vi "runtimeTest.vi"() -> ()   [LabVIEW 2017, in "JSON_RPC_Interface tests.lvlib"]
uses:
  JSON_RPC_Interface tests.lvlib
  module/execution/JSON_RPC_Interface runtime.lvclass
  <vilib>/NI/Tag Bus/dictionary/data dictionary.lvclass/data dictionary.ctl
  <vilib>/NI/Tag Bus/dictionary/lookup polymorphs/locate double.vi
  <vilib>/NI/Tag Bus/dictionary/lookup polymorphs/locate Array of String.vi
  <vilib>/NI/Tag Bus/table/data polymorphs/write one/write Double.vi
  <vilib>/NI/Tag Bus/table/data polymorphs/write one/write Array of String.vi
  <vilib>/NI/Tag Bus/table/data polymorphs/read one/read Double.vi
  <vilib>/NI/Tag Bus/table/data polymorphs/read one/read Array of String.vi
  <vilib>/NI/Tag Bus/dictionary/search/find data index.vi
  <vilib>/NI/Tag Bus/dictionary/search/search string list.vi
  module/configuration/JSON_RPC_Interface configuration.lvclass
  C:/Program Files (x86)/National Instruments/LabVIEW 2017/vi.lib/NI/Tag Bus Module Framework/module configuration/TBM module configuration.lvclass
  <vilib>/NI/Tag Bus/dictionary/tag not found.vi
  <vilib>/NI/Tag Bus/dictionary/data dictionary.lvclass
  <vilib>/NI/Tag Bus/table/data table.lvlib
panel:
  out "Input ArrayOfString":string[](array[string])
  in  "Output ArrayOfString":string[](array[string])
  in  "stop":bool
  in  "output value":dbl=42.0 format="%#_13g"
  out "Input value":dbl
  out "Names":string[](array[string])
  out "final error":errorcluster
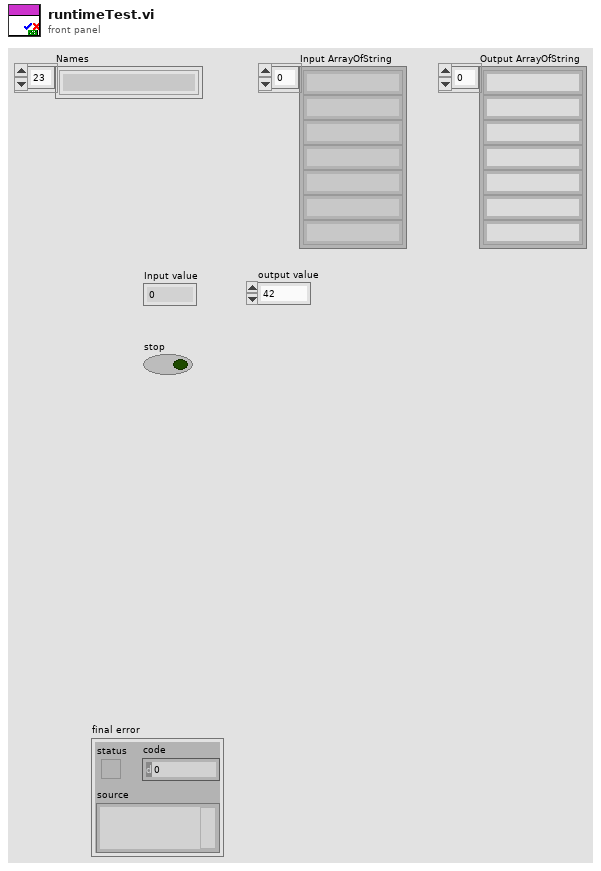
[diagram p1: front panel]
types:
  T1 = typedef "TBM channel.lvclass/data tables.ctl" = cluster{"input data":T2, "processing parameter":T2, "processing result":T2, "output data":T2}
  T2 = typedef "tag bus.lvlib/dictionary table pair.ctl" = cluster{"data dictionary":refnum<class "data dictionary.lvclass">, "data table":T3}
  T3 = typedef "tag bus.lvlib/data table.lvlib/data table.ctl" = cluster{"Double":dbl[], "Single":sgl[], "I64":i64[], "I32":i32[], "I16":i16[], "I8":i8[], "U64":u64[], "U32":u32[], "U16":u16[], "U8":u8[], "Boolean":bool[], "String":string[], "Array of Double":cluster{"DBL Array":dbl[]}[], "Array of Single":cluster{"SGL Array":sgl[]}[], "Array of I64":cluster{"I64 Array":i64[]}[], "Array of I32":cluster{"I32 Array":i32[]}[], "Array of I16":cluster{"I16 Array":i16[]}[], "Array of I8":cluster{"I8 Array":i8[]}[], "Array of U64":cluster{"U64 Array":u64[]}[], "Array of U32":cluster{"U32 Array":u32[]}[], "Array of U16":cluster{"U16 Array":u16[]}[], "Array of U8":cluster{"U8 Array":u8[]}[], "Array of Boolean":cluster{"Boolean Array":bool[]}[], "Array of String":cluster{"String Array":string[]}[]}
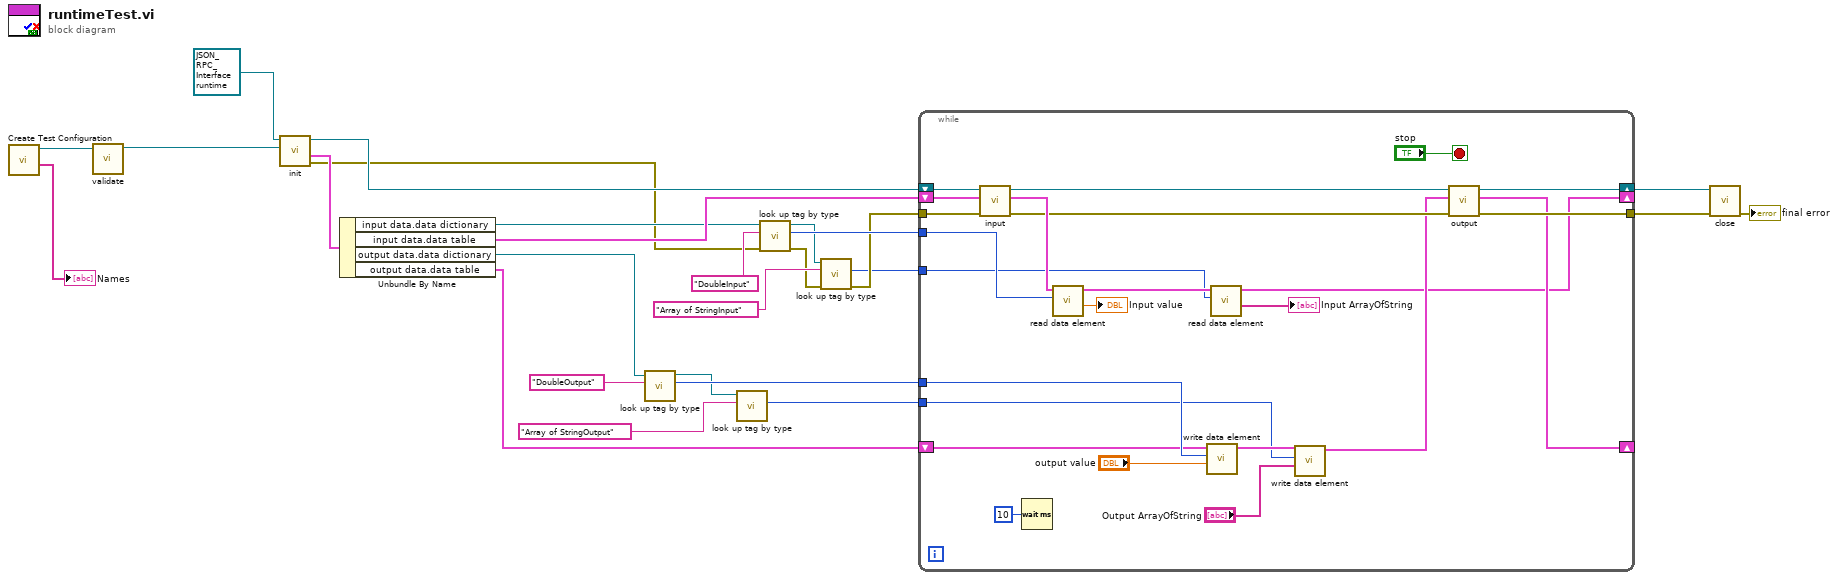
[diagram p0: block diagram]
diagram:
  n1 = call "Create Test Configuration.vi"() -> ("Names"=→"Names":string[], "Module Configuration"=w24:refnum<class "JSON_RPC_Interface configuration.lvclass">)  [unwired: 6 in, 4 out]
  n2 = call-dynamic "validate.vi"("JSON_RPC_Interface configuration in"=w24) -> ("JSON_RPC_Interface configuration out"=w25:refnum<class "JSON_RPC_Interface configuration.lvclass">)  [unwired: 9 in, 1 out]
  n3 = call-dynamic "init.vi"("TBM module configuration in"=w25, "JSON_RPC_Interface runtime in"=refnum<class "JSON_RPC_Interface runtime.lvclass"> refnum ("tag bus configurable plugin module")) -> ("error out"=w9:errorcluster, "data allocations"=w17:T1, "JSON_RPC_Interface runtime out"=w16:refnum<class "JSON_RPC_Interface runtime.lvclass">)  [unwired: 6 in, 1 out]
  n4 = Unbundle By Name(w17) -> ("input data.data dictionary"=w14:refnum<class "data dictionary.lvclass">, "input data.data table"=w15:T3, "output data.data dictionary"=w10:refnum<class "data dictionary.lvclass">, "output data.data table"=w11:T3)
  n5 = call-poly <vilib>:"look up tag by type.vi"("name"="DoubleOutput" ("channel name"), "data dictionary in"=w10) -> ("index"=w21:i32, "data dictionary out"=w4:refnum<class "data dictionary.lvclass">)  [unwired: 7 in, 1 out]
  n6 = call-poly <vilib>:"look up tag by type.vi"("name"="Array of StringOutput" ("channel name"), "data dictionary in"=w4) -> ("index"=w1:i32)  [unwired: 7 in, 2 out]
  n7 = call-poly <vilib>:"look up tag by type.vi"("error in"=w9, "name"="DoubleInput" ("channel name"), "data dictionary in"=w14) -> ("error out"=w6:errorcluster, "index"=w12:i32, "data dictionary out"=w7:refnum<class "data dictionary.lvclass">)  [unwired: 6 in]
  n8 = call-poly <vilib>:"look up tag by type.vi"("error in"=w6, "name"="Array of StringInput" ("channel name"), "data dictionary in"=w7) -> ("error out"=w5:errorcluster, "index"=w2:i32)  [unwired: 6 in, 1 out]
  n9 = while {
    tunnel: w5 -> [w50]
    tunnel: w21 -> [w48]
    tunnel: [w44] -> w19
    tunnel: w12 -> [w41]
    shift-right: [w45] -> w20
    shift-left: w16 -> [w43]
    shift-right: [w29] -> _
    shift-left: w15 -> [w42]
    shift-right: [w35] -> _
    shift-left: w11 -> [w39]
    tunnel: w2 -> [w28]
    tunnel: w1 -> [w32]
    stop <- "stop" stop-if-true
    n10 = call-dynamic "input.vi"("error in"=w50, "data table in"=w42, "JSON_RPC_Interface runtime in"=w43) -> ("error out"=w37:errorcluster, "data table out"=w49:T3, "JSON_RPC_Interface runtime out"=w46:refnum<class "JSON_RPC_Interface runtime.lvclass">)  [unwired: 6 in]
    n11 = Wait (ms)(milliseconds to wait=u32 10) -> ()  [unwired: 1 out]
    n12 = call-poly <vilib>:"read data element.vi"("index"=w41, "data table in"=w49) -> ("value"=→"Input value":dbl, "data table out"=w30:T3)  [unwired: 8 in]
    n13 = call-poly <vilib>:"write data element.vi"("value"="output value", "index"=w48, "data table in"=w39) -> ("data table out"=w34:T3)  [unwired: 8 in]
    n14 = call-poly <vilib>:"read data element.vi"("index"=w28, "data table in"=w30) -> ("value"=→"Input ArrayOfString":string[], "data table out"=w29:T3)  [unwired: 8 in]
    n15 = call-poly <vilib>:"write data element.vi"("value"="Output ArrayOfString", "index"=w32, "data table in"=w34) -> ("data table out"=w33:T3)  [unwired: 8 in]
    n16 = call-dynamic "output.vi"("error in"=w37, "data table in"=w33, "JSON_RPC_Interface runtime in"=w46) -> ("error out"=w44:errorcluster, "data table out"=w35:T3, "JSON_RPC_Interface runtime out"=w45:refnum<class "JSON_RPC_Interface runtime.lvclass">)  [unwired: 6 in]
  }
  n17 = call-dynamic "close.vi"("error in"=w19, "JSON_RPC_Interface runtime in"=w20) -> ("error out"=→"final error":errorcluster)  [unwired: 9 in]
